vi "transmitter.vi"(5 "Symbol Energy":dbl=1.0 format="%#_4p", 7 "Source Type":enum16{"Random Bits", "File"}(ring), 8 "error in (no error)":errorcluster, 9 "Sync Words":i32[](array[numeric])=[1, 1, 1, 0, 0, 1, 0], 10 "Preamble Length (bits)":u32, 11 "Modulation Parameters In":T2={"TX Parameters"={"TX Oversample Factor"=4, "TX Sample Rate"=0.0}, "TX/RX Shared Parameters"={"Modulation Type"=enum."OOK", "Packet Length"=128, "# of Iterations"=0.0, "Pulse Shaping Parameters"={"Pulse Shaping Filter"=enum."none", "Filter Length (symbols)"=32, "Filter Parameter"=0.8, "modulation type"=enum."ASK"}, "Header/Tail Control Information"={"Training Sequence Type"=enum."", "Zero Pad Length"=0.0}}}) -> (0 "error out":errorcluster, 1 "output bit stream":u8[](array[numeric]), 2 "output MT waveform":cluster{"t0":dbl, "dt":dbl, "Y":cdb[]}, 3 "Modulation Parameters Out":T1={"TX Parameters"={"TX Oversample Factor"=0, "TX Sample Rate"=0.0}, "TX/RX Shared Parameters"={"Modulation Type"=enum."OOK", "Packet Length"=0.0, "# of Iterations"=0.0, "Pulse Shaping Parameters"={"Pulse Shaping Filter"=enum."none", "Filter Length (symbols)"=0, "Filter Parameter"=0.0, "modulation type"=enum."ASK"}, "Header/Tail Control Information"={"Training Sequence Type"=enum."", "Zero Pad Length"=0.0}}}, 4 "Output Symbols":cdb[](array[numeric]))   [LabVIEW 2012]
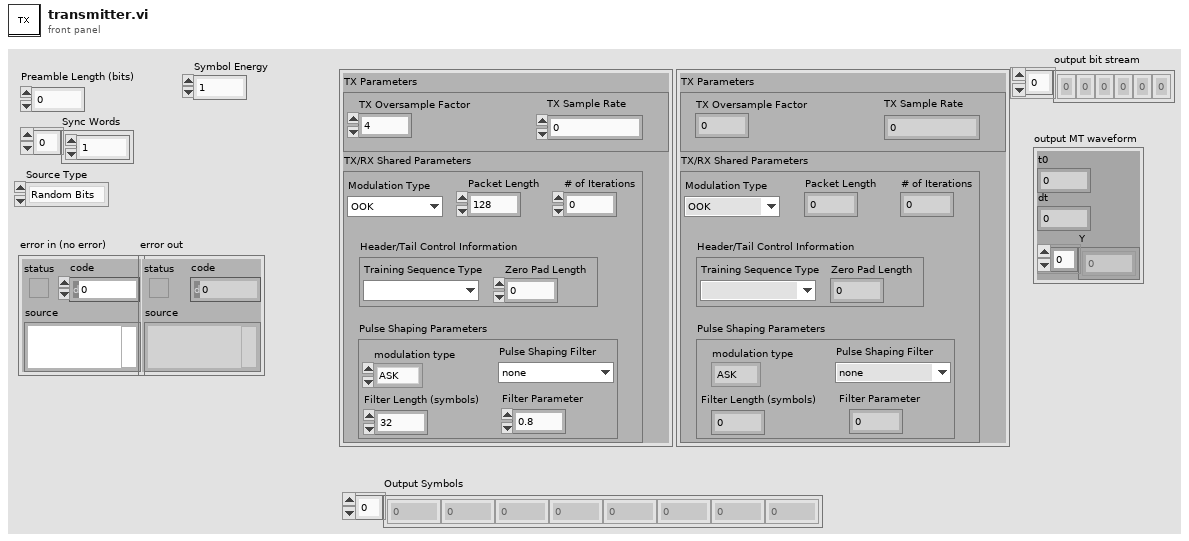
[diagram p1: front panel]
types:
  T1 = cluster{"TX Parameters":cluster{"TX Oversample Factor":i32, "TX Sample Rate":dbl}, "TX/RX Shared Parameters":cluster{"Modulation Type":enum16{"OOK", "FSK"}, "Packet Length":dbl, "# of Iterations":dbl, "Pulse Shaping Parameters":cluster{"Pulse Shaping Filter":enum16{"none", "Raised Cosine", "Root Raised Cos", "Gaussian"}, "Filter Length (symbols)":i32, "Filter Parameter":dbl, "modulation type":enum16{"FSK", "PSK", "QAM", "MSK", "PAM", "ASK", "CPM"}}, "Header/Tail Control Information":cluster{"Training Sequence Type":enum16{""}, "Zero Pad Length":dbl}}}
  T2 = cluster{"TX Parameters":cluster{"TX Oversample Factor":i32, "TX Sample Rate":dbl}, "TX/RX Shared Parameters":cluster{"Modulation Type":enum16{"OOK", "FSK"}, "Packet Length":i32, "# of Iterations":dbl, "Pulse Shaping Parameters":cluster{"Pulse Shaping Filter":enum16{"none", "Raised Cosine", "Root Raised Cos", "Gaussian"}, "Filter Length (symbols)":i32, "Filter Parameter":dbl, "modulation type":enum16{"FSK", "PSK", "QAM", "MSK", "PAM", "ASK", "CPM"}}, "Header/Tail Control Information":cluster{"Training Sequence Type":enum16{""}, "Zero Pad Length":dbl}}}
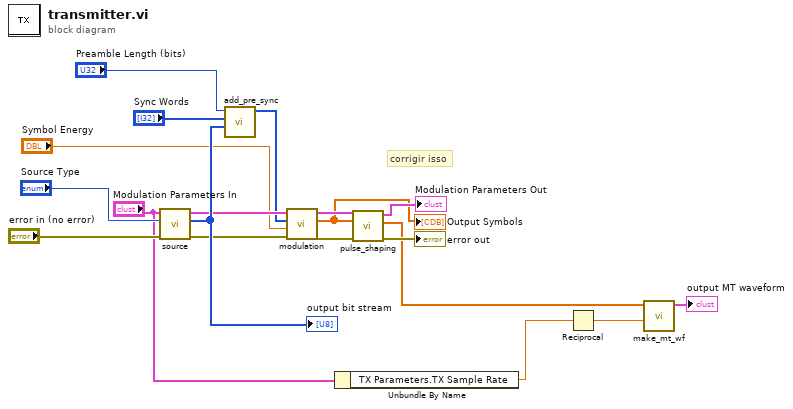
[diagram p0: block diagram]
diagram:
  # "corrigir isso"
  n1 = call "source.vi"("error in (no error)"="error in (no error)", "Type of Source"="Source Type", "Modulation Parameters In"="Modulation Parameters In") -> ("error out"=w16:errorcluster, "output bit stream"=w19:u8[], "Modulation Parameters Out"=w18:T2)  [unwired: 6 in]
  "output bit stream" <- w19
  n2 = call "add_pre_sync.vi"("Key Bit Sequence"=w19, "Sync Words"="Sync Words", "Preamble Length (bits)"="Preamble Length (bits)") -> ("Packet"=w17:i32[])  [unwired: 8 in]
  n3 = call "modulation.vi"("error in"=w16, "Symbol Energy"="Symbol Energy", "input bit stream"=w17, "Modulation Parameters In"=w18) -> ("error out"=w9:errorcluster, "Output Symbols"=w1:cdb[], "Modulation Parameters Out"=w10:T2)  [unwired: 5 in]
  "Output Symbols" <- w1
  n4 = Unbundle By Name("Modulation Parameters In") -> ("TX Parameters.TX Sample Rate"=w5:dbl)
  n5 = call "pulse_shaping.vi"("error in (no error)"=w9, "input"=w1, "Modulation Parameters In"=w10) -> ("error out"=→"error out":errorcluster, "output"=w2:cdb[], "Modulation Parameters Out"=→"Modulation Parameters Out":T2)  [unwired: 5 in, 1 out]
  n6 = Reciprocal(x=w5) -> (1/x=w4:dbl)
  n7 = call "make_mt_wf.vi"("dt"=w4, "Y"=w2) -> ("output MT waveform"=→"output MT waveform":cluster{"t0":dbl, "dt":dbl, "Y":cdb[]})  [unwired: 9 in]
